vi "Name from JSON.vi"(8 "error in (no error)":errorcluster, 10 "JSON":string, 11 "Path":path) -> (0 "error out":errorcluster, 2 "Name":string)   [LabVIEW 2023, in "VolatusSeqConfig.lvlib" / "Sequence Config.lvclass"]
uses:
  Sequence Config.lvclass
  77e003ad-7d0e-4013-b02b-912b4d5a3826.vi
  6f9d6f0a-98ce-40c0-b857-a1a217d75453.vi
  <vilib>/JDP Science/JSONtext/Next JSON Value.vi
  <vilib>/JDP Science/JSONtext/String Subset.vi
  <vilib>/JDP Science/JSONtext/Parsing/Advance past next JSON Value (inlined COPY).vi
  <vilib>/JDP Science/JSONtext/Parsing/Advance past whitespace.vi
  <vilib>/JDP Science/JSONtext/Parsing/Advance past String.vi
  <vilib>/JDP Science/JSONtext/Parsing/Advance past Number.vi
  <vilib>/JDP Science/JSONtext/Parsing/Advance past Line Ending.vi
  <vilib>/JDP Science/JSONtext/Parsing/Parse Full Path or Item Name.vi
  <vilib>/JDP Science/JSONtext/Parsing/Advance past Array.vi
  <vilib>/JDP Science/JSONtext/Parsing/Advance past Object.vi
  <vilib>/JDP Science/JSONtext/support/Error Cluster From Code.vi
  <vilib>/JDP Science/JSONtext/Offset/Find Item Locations by Path.vi
  <vilib>/JDP Science/JSONtext/JSON text to Variant.vi
  <vilib>/JDP Science/JSONtext/LVClass Serializer/JSONtext LVClass Serializer.lvclass
  Sequence Config.lvclass/Sequence Config.ctl
  <vilib>/JDP Science/JSONtext/JSONtext.lvlib
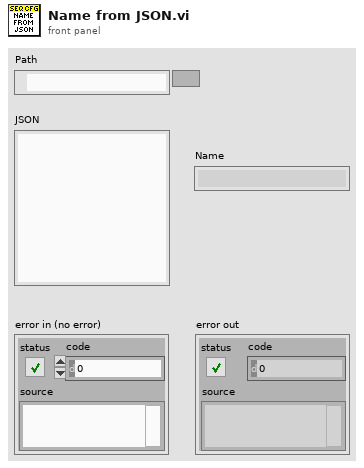
[diagram p1: front panel]
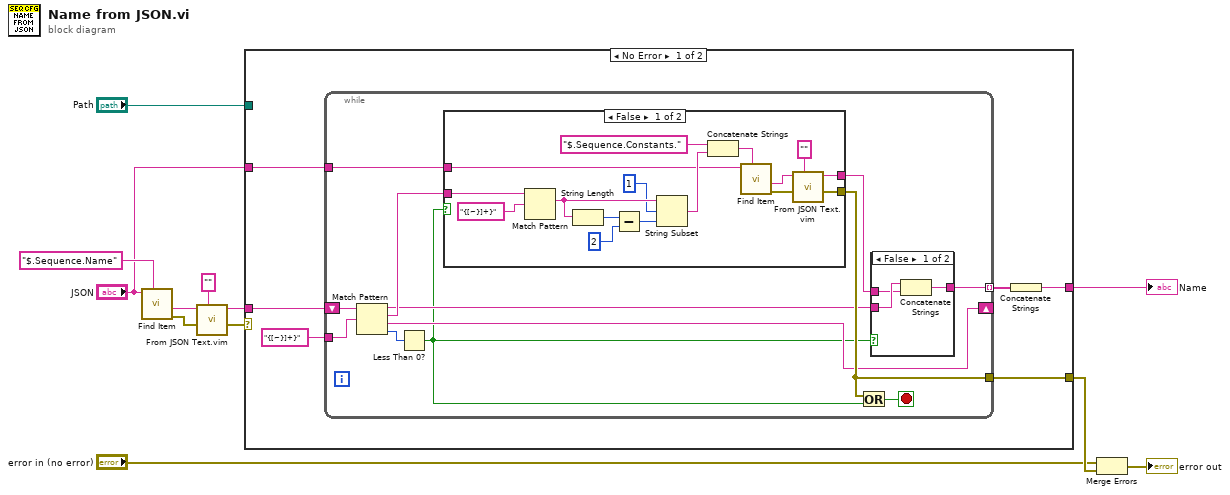
[diagram p0: block diagram]
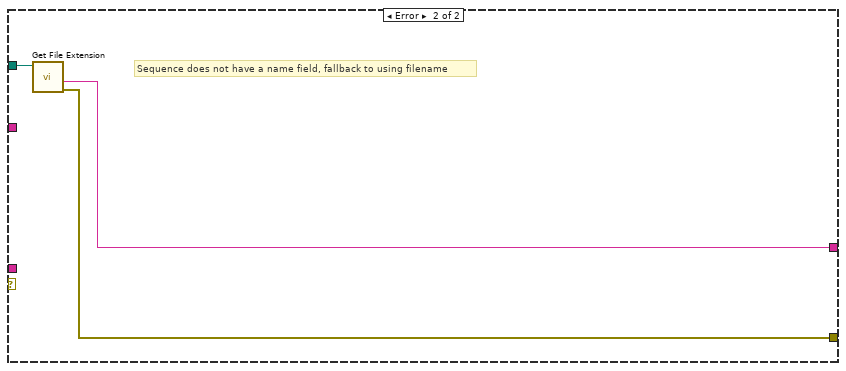
[diagram p4: hidden frame]
diagram:
  n1 = call <vilib>:"Find Item.vi"("$Path or Item Name"="$.Sequence.Name", "JSON"="JSON") -> ("error out"=w9:errorcluster, "<JSON>"=w12:string)  [unwired: 6 in, 2 out]
  n2 = call "From JSON Text.vim"("Data Type and Default Value"="", "error in (no error)"=w9, "JSON"=w12) -> ("error out"=w5:errorcluster, "Data out"=w8:string)  [unwired: 7 in]
  n3 = case shown="No Error" w5 {
    tunnel: w8 -> [w17 _]
    tunnel: "JSON" -> [w16 _]
    tunnel: [w14 w52] -> w6
    tunnel: [w13 w51] -> w3
    tunnel: "Path" -> [_ w53]
    frame No Error {
      n4 = while {
        shift-right: [w22] -> _
        shift-left: w17 -> [w29]
        tunnel: "{[~}]+}" ("regular expression") -> [w28]
        tunnel: [w30] -> w13
        tunnel: [w21] -> w15 mode=indexing
        tunnel: w16 -> [w20]
        stop <- w24 stop-if-true
        n5 = Match Pattern(string=w29, regular expression=w28) -> (before substring=w23:string, match substring=w27:string, after substring=w22:string, offset past match=w26:i32)  [unwired: 1 in]
        n6 = Less Than 0?(x=w26) -> (x < 0?=w19:bool)
        n7 = case shown="False" w19 {
          tunnel: w27 -> [w40 _]
          tunnel: [w32 _] -> w25
          tunnel: w20 -> [w37 _]
          tunnel: [w31 _] -> w30
          frame False {
            n8 = Match Pattern(string=w40, regular expression="{[~}]+}") -> (match substring=w43:string)  [unwired: 1 in, 3 out]
            n9 = String Length(string=w43) -> (length=w45:i32)
            n10 = Subtract(x=w45, y=2) -> (x-y=w42:i32)
            n11 = String Subset(string=w43, offset (0)=1, length (rest)=w42) -> (substring=w38:string)
            n12 = Concatenate Strings("$.Sequence.Constants.", w38) -> (w36:string)
            n13 = call <vilib>:"Find Item.vi"("$Path or Item Name"=w36, "JSON"=w37) -> ("error out"=w33:errorcluster, "<JSON>"=w34:string)  [unwired: 6 in, 2 out]
            n14 = call "From JSON Text.vim"("Data Type and Default Value"="", "error in (no error)"=w33, "JSON"=w34) -> ("error out"=w31:errorcluster, "Data out"=w32:string)  [unwired: 7 in]
          }
          frame True {
          }
        }
        n15 = Or(x=w30, y=w19) -> (x .or. y?=w24:bool)
        n16 = case shown="False" w19 {
          tunnel: w23 -> [w49 w50]
          tunnel: w25 -> [w47 _]
          tunnel: [w48 w50] -> w21
          frame False {
            n17 = Concatenate Strings(w49, w47) -> (w48:string)
          }
          frame True {
          }
        }
      }
      n18 = Concatenate Strings(w15) -> (w14:string)
    }
    frame Error {
      # "Sequence does not have a name field, fallback to using filename"
      n19 = call <vilib>:"Get File Extension.vi"("file"=w53) -> ("error out"=w51:errorcluster, "filename without extension"=w52:string)  [unwired: 6 in, 3 out]
    }
  }
  "Name" <- w6
  n20 = Merge Errors("error in (no error)", w3) -> (→"error out":errorcluster)
